vi "Auto Gear Align (2).vi"(8 "Error In":errorcluster, 9 "R/G/B":cluster{"Lower value":i32, "Upper value":i32}[](array[cluster])=[{"Lower value"=0, "Upper value"=40}, {"Lower value"=80, "Upper value"=255}, {"Lower value"=0, "Upper value"=255}], 10 "Camera Image":T2, 11 "Refnum's In":T1={"RobotDrive"="RobotDrive", "Gyro"="Gyro", "Mtr 1"="LeftMtr", "Mtr 2"="RightMtr"}) -> (0 "Error Out":errorcluster, 3 "Refnum's Out":T1={"RobotDrive"="RobotDrive", "Gyro"="Gyro", "Mtr 1"="LeftMtr", "Mtr 2"="RightMtr"})   [LabVIEW 2016]
uses:
  <vilib>/vision/Image Controls.llb/IMAQ Image.ctl
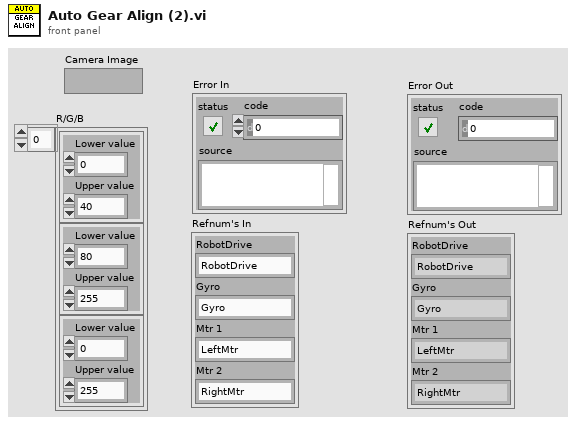
[diagram p1: front panel]
types:
  T1 = cluster{"RobotDrive":string, "Gyro":string, "Mtr 1":string, "Mtr 2":string}
  T2 = typedef "IMAQ Image.ctl" = refnum<image>
  T3 = cluster{"Left":dbl, "Top":dbl, "Right":dbl, "Bottom":dbl}
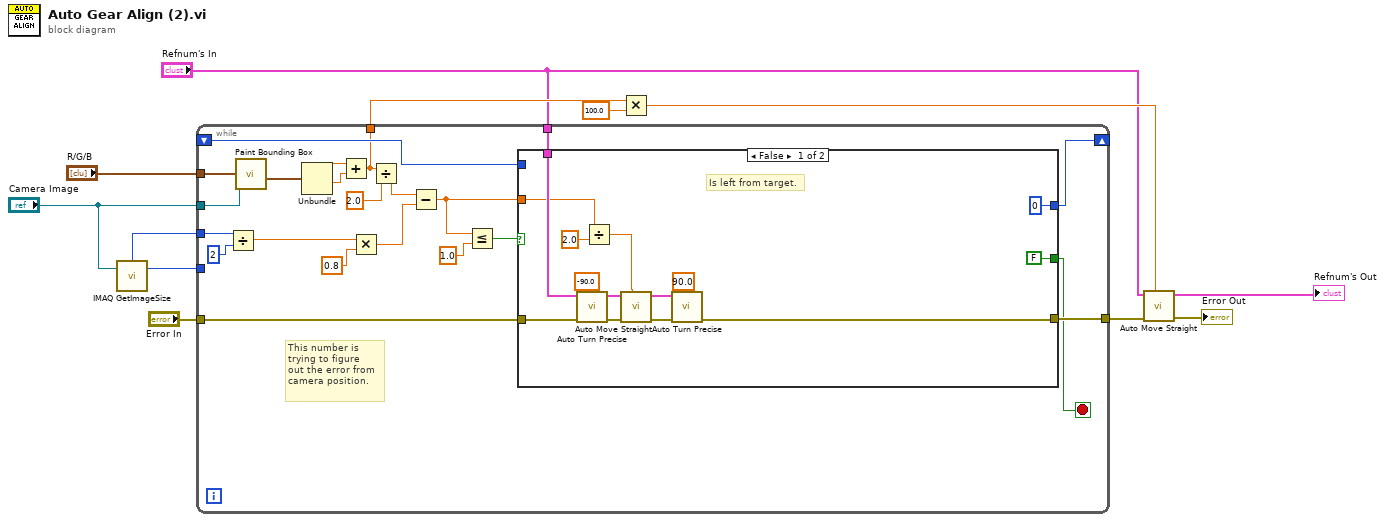
[diagram p0: block diagram]
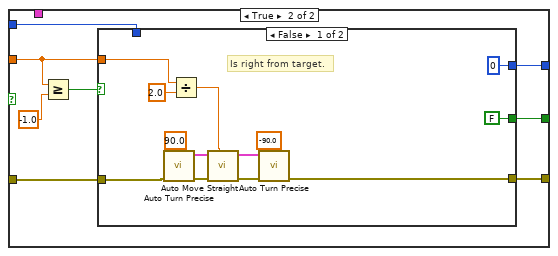
[diagram p2: hidden frame]
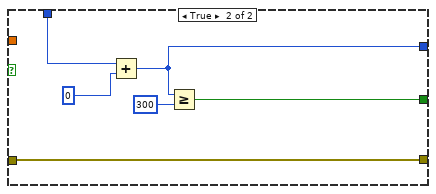
[diagram p3: hidden frame]
diagram:
  n1 = call "IMAQ GetImageSize"("Image"="Camera Image") -> ("Y Resolution"=w10:i32, "X Resolution"=w9:i32)  [unwired: 3 in, 1 out]
  n2 = while {
    tunnel: "Camera Image" -> [w34]
    tunnel: "R/G/B" -> [w33]
    tunnel: w10 -> [_]
    tunnel: w9 -> [w31]
    tunnel: "Refnum's In" -> [w24]
    shift-right: [w18] -> _
    shift-left: _ -> [w17]
    tunnel: [w16] -> w8
    tunnel: "Error In" -> [w15]
    tunnel: [w14] -> w3
    stop <- w13 stop-if-true
    # "This number is \ntrying to figure\nout the error from\ncamera position."
    n3 = Divide(x=w31, y=2) -> (x/y=w29:dbl)
    n4 = call "Paint Bounding Box.vi"("Camera Image"=w34, "R/G/B"=w33) -> ("Bounding Box Final"=w32:T3)  [unwired: 5 in, 4 out]
    n5 = Unbundle(w32) -> ("Left"=w27:dbl, "Right"=w26:dbl)  [unwired: 2 out]
    n6 = Add(x=w27, y=w26) -> (x+y=w16:dbl)
    n7 = Multiply(x=w29, y=0.8) -> (x*y=w22:dbl)
    n8 = Divide(x=w16, y=2.0) -> (x/y=w23:dbl)
    n9 = Subtract(x=w23, y=w22) -> (x-y=w20:dbl)
    n10 = Less Or Equal?(x=w20, y=1.0) -> (x <= y?=w21:bool)
    n11 = case shown="False" w21 {
      tunnel: w24 -> [w48 _]
      tunnel: w20 -> [w44 w54]
      tunnel: [0 w53] -> w18
      tunnel: w17 -> [_ w52]
      tunnel: [FALSE w51] -> w13
      tunnel: w15 -> [w36 w50]
      tunnel: [w35 w49] -> w14
      frame False {
        # "Is left from target."
        n12 = call "Auto Turn Precise.vi"("Target Distance"=-90.0, "Error In"=w36, "Refnum's In"=w48) -> ("Error Out"=w46:errorcluster, "Refnum's Out"=w45:T1)  [unwired: 7 in]
        n13 = Divide(x=w44, y=2.0) -> (x/y=w42:dbl)
        n14 = call "Auto Move Straight.vi"("Target Distance"=w42, "Error In"=w46, "Refnum's In"=w45) -> ("Error Out"=w40:errorcluster, "Refnum's Out"=w39:T1)  [unwired: 7 in]
        n15 = call "Auto Turn Precise.vi"("Target Distance"=90.0, "Error In"=w40, "Refnum's In"=w39) -> ("Error Out"=w35:errorcluster)  [unwired: 7 in, 1 out]
      }
      frame True {
        n16 = Greater Or Equal?(x=w54, y=-1.0) -> (x >= y?=w55:bool)
        n17 = case shown="False" w55 {
          tunnel: w54 -> [w61 _]
          tunnel: w52 -> [_ w75]
          tunnel: [0 w72] -> w53
          tunnel: [FALSE w71] -> w51
          tunnel: w50 -> [w58 w70]
          tunnel: [w57 w70] -> w49
          frame False {
            # "Is right from target."
            n18 = call "Auto Turn Precise.vi"("Target Distance"=90.0, "Error In"=w58) -> ("Error Out"=w68:errorcluster, "Refnum's Out"=w67:T1)  [unwired: 8 in]
            n19 = Divide(x=w61, y=2.0) -> (x/y=w65:dbl)
            n20 = call "Auto Move Straight.vi"("Target Distance"=w65, "Error In"=w68, "Refnum's In"=w67) -> ("Error Out"=w63:errorcluster, "Refnum's Out"=w62:T1)  [unwired: 7 in]
            n21 = call "Auto Turn Precise.vi"("Target Distance"=-90.0, "Error In"=w63, "Refnum's In"=w62) -> ("Error Out"=w57:errorcluster)  [unwired: 7 in, 1 out]
          }
          frame True {
            n22 = Add(x=w75, y=0) -> (x+y=w72:i32)
            n23 = Greater Or Equal?(x=w72, y=300) -> (x >= y?=w71:bool)
          }
        }
      }
    }
  }
  n24 = Multiply(x=w8, y=100.0) -> (x*y=w6:dbl)
  n25 = call "Auto Move Straight.vi"("Target Distance"=w6, "Error In"=w3, "Refnum's In"="Refnum's In") -> ("Error Out"=→"Error Out":errorcluster, "Refnum's Out"=→"Refnum's Out":T1)  [unwired: 7 in]
